vi "Nmea Signal Divider.vi"(2 "NMEA in":string) -> (0 "Satelites":i8=-1, 1 "Fix quality":i8=-1)   [LabVIEW 2016]
uses:
  Global Variables/UTC Timestamp.vi
  Global Variables/GPS Position.vi
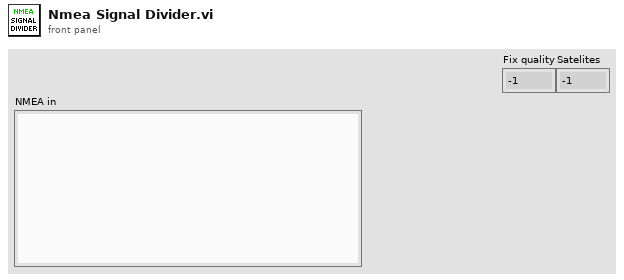
[diagram p1: front panel]
types:
  T1 = enum16{"insertPPS", "insertUTC", "read", "initiate"}
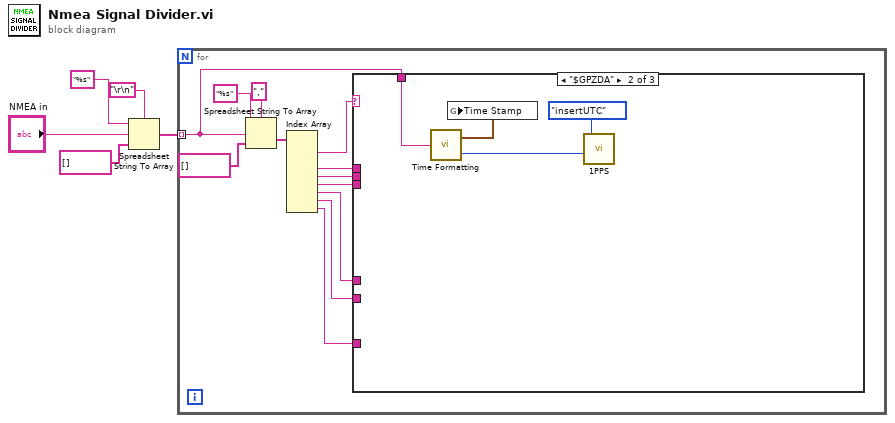
[diagram p0: block diagram]
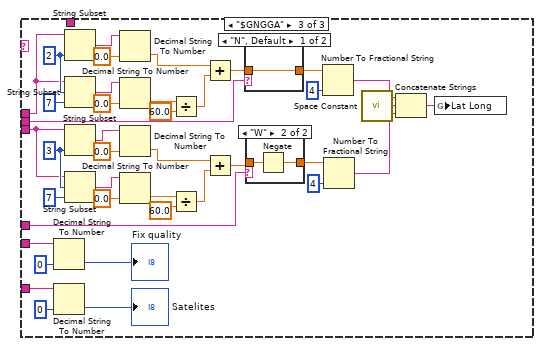
[diagram p3: hidden frame]
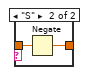
[diagram p5: hidden frame]
diagram:
  n1 = Spreadsheet String To Array(delimiter (Tab)="\r\n", format string="%s", spreadsheet string="NMEA in", array type (2D Dbl)=string[] []) -> (array=w2:string[])
  n2 = for {
    tunnel: w2 -> [w12] mode=indexing
    n3 = Spreadsheet String To Array(delimiter (Tab)="," ("search string/char (-)"), format string="%s", spreadsheet string=w12, array type (2D Dbl)=string[] []) -> (array=w14:string[])
    n4 = Index Array(array=w14) -> (element #1=w13:string, element #3=w11:string, element #4=w9:string, element #5=w10:string, element #6=w8:string, element #7=w7:string, element #8=w6:string)  [unwired: 8 in, 1 out]
    n5 = case shown="\"$GPZDA\"" w13 {
      tunnel: w12 -> [_ w18 _]
      tunnel: w11 -> [_ _ w43]
      tunnel: w10 -> [_ _ w41]
      tunnel: w9 -> [_ _ w39]
      tunnel: w8 -> [_ _ w37]
      tunnel: w7 -> [_ _ w27]
      tunnel: w6 -> [_ _ w24]
      frame Default {
      }
      frame "$GPZDA" {
        n6 = call "Time Formatting.vi"("NMEA Input"=w18) -> ("GPS UTC"=w20:timestamp, "UNIX Timestamp"=w21:u32)
        n7 = global write "UTC Timestamp.vi" "Time Stamp"(w20) -> ()
        n8 = call "1PPS.vi"("UTC ts"=w21, "Action"=T1."insertUTC") -> ()  [unwired: 2 in, 1 out]
      }
      frame "$GNGGA" {
        w47 = 3 ("length (rest)")
        w56 = 2 ("length (rest)")
        n9 = Decimal String To Number(string=w27, default (0L)=i8 0 ("default (0 I32)")) -> (number=→"Fix quality":i8)  [unwired: 1 in, 1 out]
        n10 = Decimal String To Number(string=w24, default (0L)=i8 0 ("default (0 I32)")) -> (number=→"Satelites":i8)  [unwired: 1 in, 1 out]
        n11 = String Subset(string=w43, length (rest)=w56) -> (substring=w61:string)  [unwired: 1 in]
        n12 = String Subset(string=w43, offset (0)=w56, length (rest)=7 ("length (rest)")) -> (substring=w58:string)
        n13 = String Subset(string=w41, length (rest)=w47) -> (substring=w42:string)  [unwired: 1 in]
        n14 = String Subset(string=w41, offset (0)=w47, length (rest)=7 ("length (rest)")) -> (substring=w46:string)
        n15 = Decimal String To Number(string=w61, default (0L)=0.0 ("default (0 I32)")) -> (number=w52:dbl)  [unwired: 1 in, 1 out]
        n16 = Decimal String To Number(string=w58, default (0L)=0.0 ("default (0 I32)")) -> (number=w55:dbl)  [unwired: 1 in, 1 out]
        n17 = Decimal String To Number(string=w42, default (0L)=0.0 ("default (0 I32)")) -> (number=w51:dbl)  [unwired: 1 in, 1 out]
        n18 = Decimal String To Number(string=w46, default (0L)=0.0 ("default (0 I32)")) -> (number=w48:dbl)  [unwired: 1 in, 1 out]
        n19 = Divide(x=w55, y=60.0) -> (x/y=w53:dbl)
        n20 = Divide(x=w48, y=60.0) -> (x/y=w50:dbl)
        n21 = Add(x=w52, y=w53) -> (x+y=w40:dbl)
        n22 = Add(x=w51, y=w50) -> (x+y=w38:dbl)
        n23 = case shown="\"N\", Default" w39 {
          tunnel: w40 -> [w65 w67]
          tunnel: [w65 w66] -> w36
          frame "N", Default {
          }
          frame "S" {
            n24 = Negate(x=w67) -> (-x=w66:dbl)
          }
        }
        n25 = case shown="\"W\"" w37 {
          tunnel: w38 -> [w62 w64]
          tunnel: [w62 w63] -> w33
          frame "E", Default {
          }
          frame "W" {
            n26 = Negate(x=w64) -> (-x=w63:dbl)
          }
        }
        n27 = Number To Fractional String(number=w36, precision (6)=i16 4) -> (F-format string=w32:string)  [unwired: 2 in]
        n28 = Number To Fractional String(number=w33, precision (6)=i16 4) -> (F-format string=w31:string)  [unwired: 2 in]
        n29 = call <vilib>:"Space Constant.vi"() -> ("String"=w30:string)
        n30 = Concatenate Strings(w32, w30, w31) -> (w29:string)
        n31 = global write "GPS Position.vi" "Lat Long"(w29) -> ()
      }
    }
  }
